vi "Close JSON Config File.vi"(8 "error in (no error)":errorcluster, 11 "JSON Config File in":refnum<class "JSON Config File.lvclass">) -> (0 "error out":errorcluster)   [LabVIEW 2013, in "JSON Config File.lvclass"]
uses:
  JSON Config File.lvclass
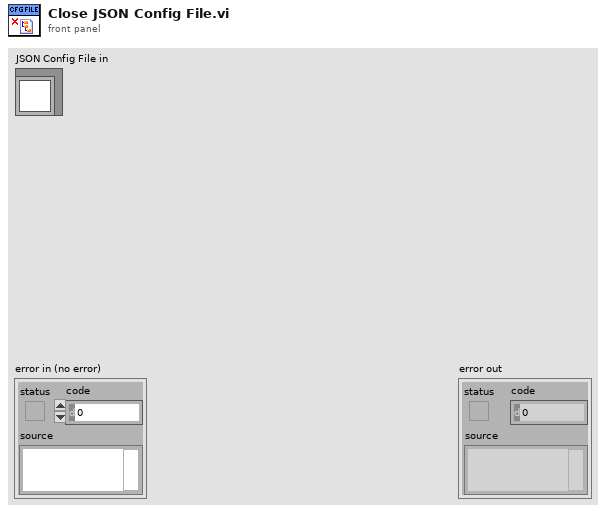
[diagram p1: front panel]
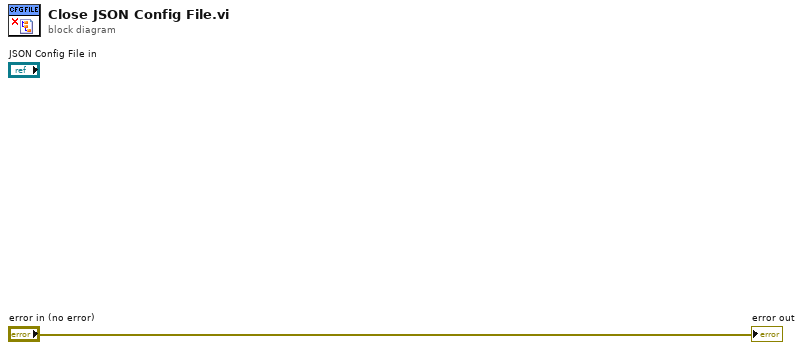
[diagram p0: block diagram]
diagram:
  "error out" <- "error in (no error)"
